vi "Init Module.vi"(8 "error in (no error)":errorcluster, 10 "Close Master Reference (F)":bool, 11 "Cloneable Module Admin in":refnum<class "Delacor_lib_QMH_Cloneable Module Admin.lvclass">) -> (0 "error out":errorcluster, 2 "GenNet-Client Request Events":T1, 3 "Cloneable Module Admin out":refnum<class "Delacor_lib_QMH_Cloneable Module Admin.lvclass">)   [LabVIEW 2022 SP3, in "GenNet-Client.lvlib"]
doc: "Initialize the module by creating Broadcast Events, Request Events, and synchronization rendezvous. Also, since this is a cloneable module, add it to the cloneable registry and update the Module Admin class.\n____\nHAMPEL SOFTWARE ENGINEERING v3.8.0 (2023-12-18 14:41)"
uses:
  GenNet-Client.lvlib
  <vilib>/Delacor/Delacor QMH/Libraries/Cloneable Module Admin_class/Delacor_lib_QMH_Cloneable Module Admin.lvclass
  C:/Program Files/National Instruments/LabVIEW 2022/vi.lib/Delacor/Delacor QMH/Libraries/Module Admin_class/Delacor_lib_QMH_Module Admin.lvclass
  Request Events--cluster.ctl
  Stop Argument--cluster.ctl
  Show Panel Argument--cluster.ctl
  Hide Panel Argument--cluster.ctl
  Show Diagram Argument--cluster.ctl
  Get Module Execution Status Argument--cluster.ctl
  Send via Network Argument--cluster.ctl
  Connect Argument--cluster.ctl
  Connect (Reply Payload)--cluster.ctl
  Listen for Network Broadcasts Argument--cluster.ctl
  <vilib>/Delacor/Delacor QMH/Libraries/Module Admin_class/Delacor_lib_QMH_Module Admin.lvclass/Delacor_lib_QMH_Module Admin.ctl
  <vilib>/Delacor/Delacor QMH/Libraries/Cloneable Module Admin_class/Delacor_lib_QMH_Cloneable Module Admin.lvclass/Delacor_lib_QMH_Cloneable Module Admin.ctl
  <vilib>/Delacor/Delacor QMH/Libraries/Module Admin_class/Delacor_lib_QMH_Get External Launch.vi
  <vilib>/Delacor/Delacor QMH/Libraries/Cloneable Module Admin_class/Delacor_lib_QMH_Get Module ID.vi
  <vilib>/Delacor/Delacor QMH/Libraries/Cloneable Module Admin_class/Delacor_lib_QMH_Set Close Master Reference.vi
  <vilib>/Delacor/Delacor QMH/Libraries/Cloneable Module Admin_class/Delacor_lib_QMH_Set First.vi
  Clone Registration/Clone Registration.lvlib
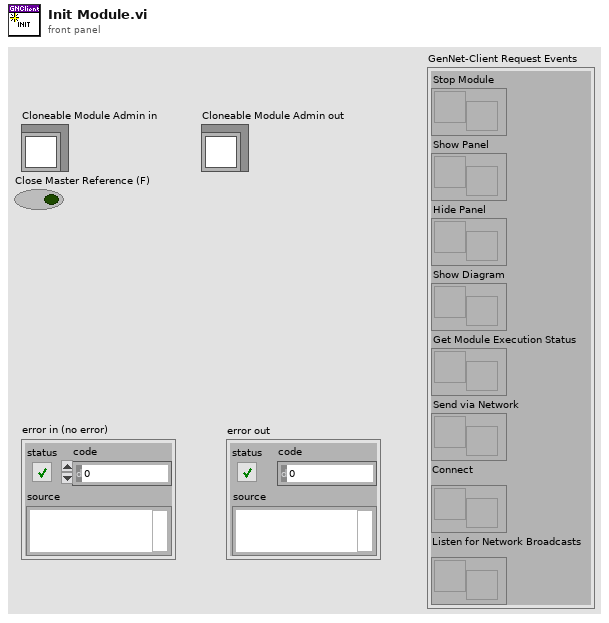
[diagram p1: front panel]
types:
  T1 = typedef "GenNet-Client.lvlib/Request Events--cluster.ctl" = cluster{"Stop Module":refnum<user-event>, "Show Panel":refnum<user-event>, "Hide Panel":refnum<user-event>, "Show Diagram":refnum<user-event>, "Get Module Execution Status":refnum<user-event>, "Send via Network":refnum<user-event>, "Connect":refnum<user-event>, "Listen for Network Broadcasts":refnum<user-event>}
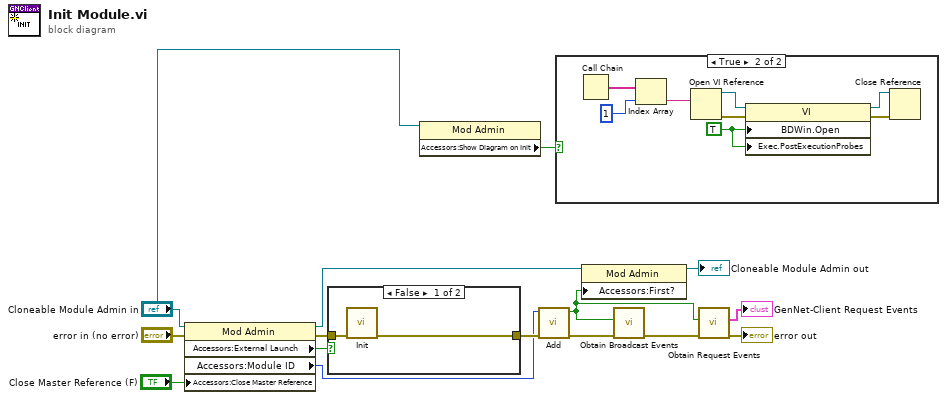
[diagram p0: block diagram]
diagram:
  n1 = property class="Mod Admin"(reference="Cloneable Module Admin in", error in="error in (no error)", "Accessors:Close Master Reference"="Close Master Reference (F)") -> (reference out=w9:refnum<class "Delacor_lib_QMH_Cloneable Module Admin.lvclass">, error out=w4:errorcluster, "Accessors:External Launch"=w8:bool, "Accessors:Module ID"=w3:i32)
  n2 = case "External Launch?" shown="False" w8 {
    tunnel: [w17 w18] -> w14
    tunnel: w4 -> [w16 w18]
    frame False {
      n3 = call "Init.vi"("error in (no error)"=w16) -> ("error out"=w17:errorcluster)  [unwired: 7 in, 3 out]
    }
    frame True {
      # "Init of Clone's registration\nhappened at Start Module.vi"
    }
  }
  n4 = property class="Mod Admin"(reference="Cloneable Module Admin in") -> ("Accessors:Show Diagram on Init"=w1:bool)  [unwired: 1 in, 2 out]
  n5 = call "Add.vi"("error in (no error)"=w14, "Module ID"=w3) -> ("error out"=w15:errorcluster, "First?"=w10:bool)  [unwired: 7 in, 1 out]
  n6 = case shown="True" w1 {
    frame False {
    }
    frame True {
      w22 = TRUE ("Block Diagram Window:Open")
      n7 = Call Chain() -> (call chain=w26:string[])
      n8 = Index Array(array=w26, index=1) -> (element=w19:string)
      n9 = Open VI Reference(vi path=w19) -> (vi reference=w23:refnum<vi>, error out=w24:errorcluster)  [unwired: 5 in]
      n10 = property class="VI"(reference=w23, error in=w24, "BDWin.Open"=w22, "Exec.PostExecutionProbes"=w22) -> (reference out=w20:refnum<vi>, error out=w21:errorcluster)
      n11 = Close Reference(reference=w20, error in (no error)=w21) -> ()  [unwired: 1 out]
    }
  }
  n12 = property class="Mod Admin"(reference=w9, "Accessors:First?"=w10) -> (reference out=→"Cloneable Module Admin out":refnum<class "Delacor_lib_QMH_Cloneable Module Admin.lvclass">)  [unwired: 1 in, 1 out]
  n13 = call "Obtain Broadcast Events.vi"("error in (no error)"=w15, "Create New?"=w10) -> ("error out"=w13:errorcluster)  [unwired: 8 in, 1 out]
  n14 = call "Obtain Request Events.vi"("error in (no error)"=w13, "Create New?"=w10) -> ("error out"=→"error out":errorcluster, "GenNet-Client Request Events"=→"GenNet-Client Request Events":T1)  [unwired: 8 in]
